vi "ModeChange.vi"(6 "DB":T1 items=["Server", "Local DB"], 7 "References":T2, 8 "error in":errorcluster, 9 "Ctrl in":refnum<vi>, 10 "Mode in":T12, 11 "Queues in":T9) -> (0 "error out":errorcluster, 2 "Mode out":T12, 3 "Queues out":T9)   [LabVIEW 2019]
uses:
  TypeDef/#TypeDef_Enum_Buttons.ctl
  Queue/TypeDef/#TypeDef_App_Queues.ctl
  TypeDef/#TypeDef_EventStructureConstant.ctl
  TypeDef/#TypeDef_Enum_EventStructure.ctl
  Queue/TypeDef/#TypeDef_NetworkStream.ctl
  Communication/TypeDef/#TypeDef_FromMRtoPC.ctl
  Communication/TypeDef/#TypeDef_FromPCtoMR.ctl
  Communication/TypeDef/#TypeDef_Command.ctl
  Communication/TypeDef/#TypeDef_ErrorHandler_prop.ctl
  Communication/TypeDef/#TypeDef_PropGraph.ctl
  Communication/TypeDef/#TypeDef_PropertiesToSave.ctl
  <vilib>/addons/database/Connection.llb/Conn ObjectReference.ctl
  Test/TypeDef/#TypeDef_DataToTest.ctl
  TypeDef/#TypeDef_References.ctl
  TypeDef/#TypeDef_Buttons.ctl
  TypeDef/#TypeDef_ReferencesMeassurementProp.ctl
  TypeDef/#TypeDef_ReferencesArchiveProp.ctl
  TypeDef/#TypeDef_Lists.ctl
  TypeDef/#TypeDef_MeasProp.ctl
  TypeDef/#TypeDef_OpProp.ctl
  TypeDef/#TypeDef_Enum_ModeOp.ctl
  Data Saving/DataBase/TypeDef/#TypeDef_DBMode.ctl
  <vilib>/addons/database/NI_Database_API.lvlib
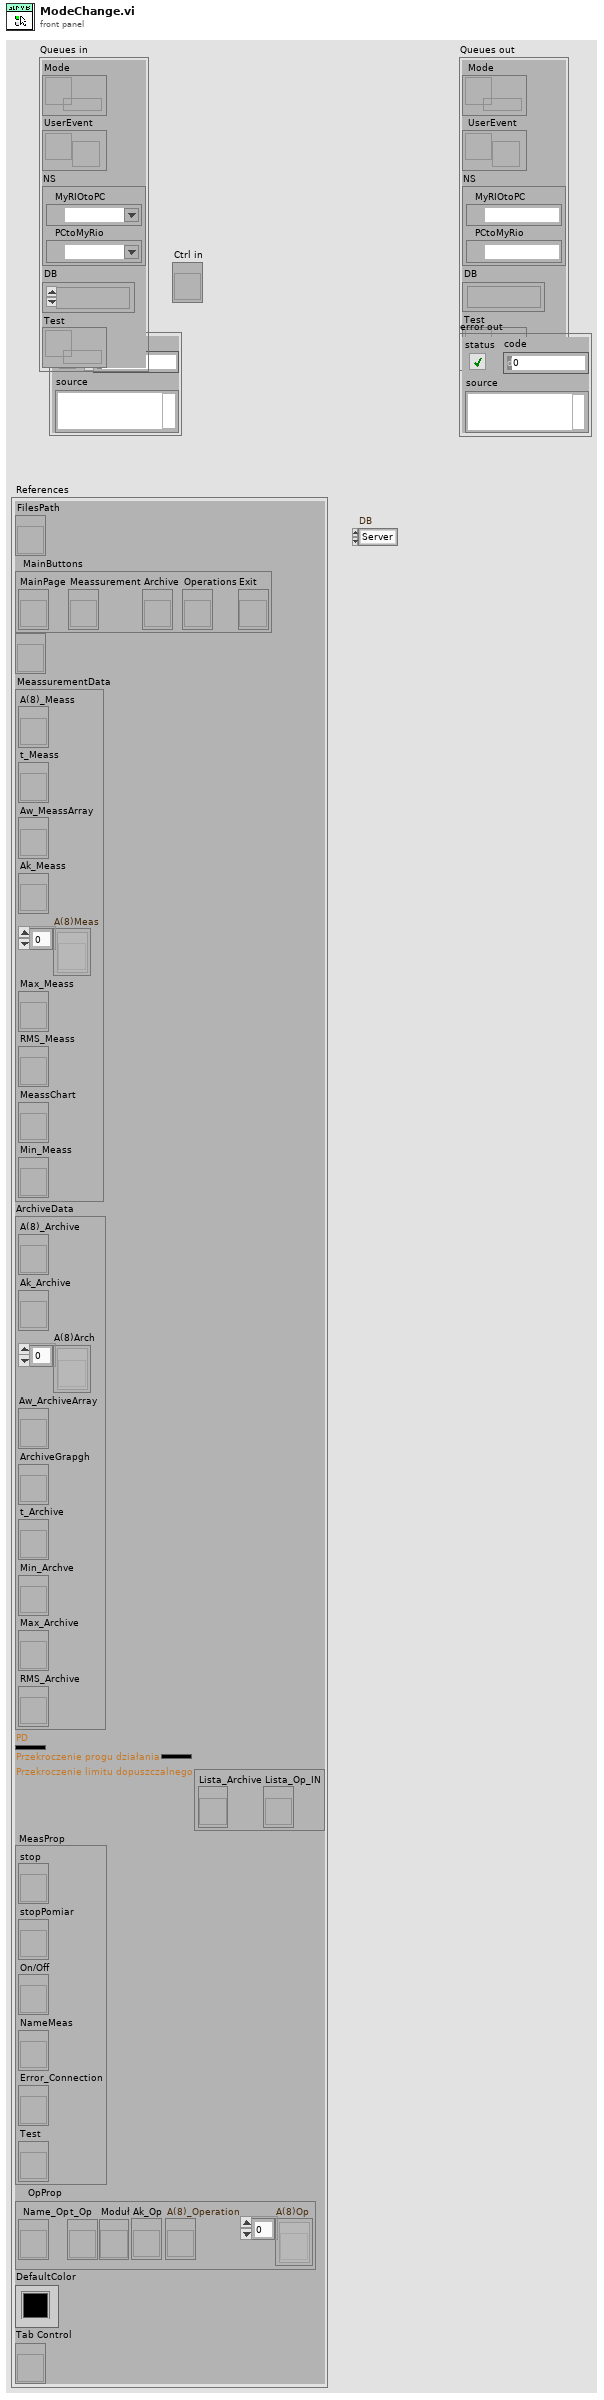
[diagram p1: front panel]
types:
  T1 = typedef "#TypeDef_DBMode.ctl" = u16
  T2 = typedef "#TypeDef_References.ctl" = cluster{"FilesPath":refnum<vi>, "MainButtons":T3, "Lista CTRL":refnum<vi>, "MeassurementData":T4, "ArchiveData":T5, "PD":u32, "LD":u32, "Lists":T6, "MeasProp":T7, "OpProp":T8, "DefaultColor":u32, "Tab Control":refnum<vi>}
  T3 = typedef "#TypeDef_Buttons.ctl" = cluster{"MainPage":refnum<vi>, "Meassurement":refnum<vi>, "Archive":refnum<vi>, "Operations":refnum<vi>, "Exit":refnum<vi>}
  T4 = typedef "#TypeDef_ReferencesMeassurementProp.ctl" = cluster{"A(8)_Meass":refnum<vi>, "t_Meass":refnum<vi>, "Aw_MeassArray":refnum<vi>, "Ak_Meass":refnum<vi>, "A(8)Meas":refnum<vi>[], "Max_Meass":refnum<vi>, "RMS_Meass":refnum<vi>, "MeassChart":refnum<vi>, "Min_Meass":refnum<vi>}
  T5 = typedef "#TypeDef_ReferencesArchiveProp.ctl" = cluster{"A(8)_Archive":refnum<vi>, "Ak_Archive":refnum<vi>, "A(8)Arch":refnum<vi>[], "Aw_ArchiveArray":refnum<vi>, "ArchiveGrapgh":refnum<vi>, "t_Archive":refnum<vi>, "Min_Archve":refnum<vi>, "Max_Archive":refnum<vi>, "RMS_Archive":refnum<vi>}
  T6 = typedef "#TypeDef_Lists.ctl" = cluster{"Lista_Archive":refnum<vi>, "Lista_Op_IN":refnum<vi>}
  T7 = typedef "#TypeDef_MeasProp.ctl" = cluster{"stop":refnum<vi>, "stopPomiar":refnum<vi>, "On/Off":refnum<vi>, "NameMeas":refnum<vi>, "Error_Connection":refnum<vi>, "Test":refnum<vi>}
  T8 = typedef "#TypeDef_OpProp.ctl" = cluster{"Name_Op":refnum<vi>, "t_Op":refnum<vi>, "Modu³":refnum<vi>, "Ak_Op":refnum<vi>, "A(8)_Operation":refnum<vi>, "A(8)Op":refnum<vi>[]}
  T9 = typedef "#TypeDef_App_Queues.ctl" = cluster{"Mode":refnum<queue>, "UserEvent":refnum<user-event>, "NS":T10, "DB":T11, "Test":refnum<queue>}
  T10 = typedef "#TypeDef_NetworkStream.ctl" = cluster{"MyRIOtoPC":refnum<k21>, "PCtoMyRio":refnum<k21>}
  T11 = typedef "NI_Database_API.lvlib/Conn ObjectReference.ctl" = refnum<k1>
  T12 = typedef "#TypeDef_Enum_Buttons.ctl" = enum32{"MainPage", "Pomiar", "Archiwum", "Operacje", "Wyjœcie"}
  T13 = typedef "#TypeDef_Enum_ModeOp.ctl" = enum16{"Oblicz ekspozycjê dzienn¹", "Uœrednij"}
  T14 = enum8{"Enabled", "Disabled", "Disabled and Grayed Out"}
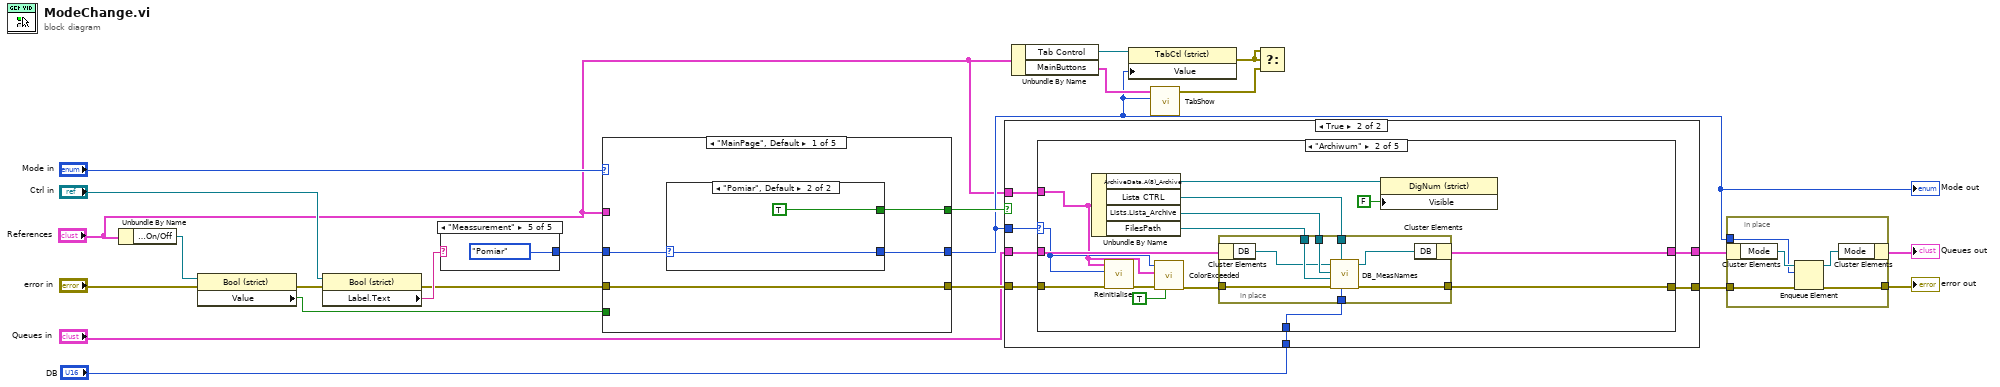
[diagram p0: block diagram]
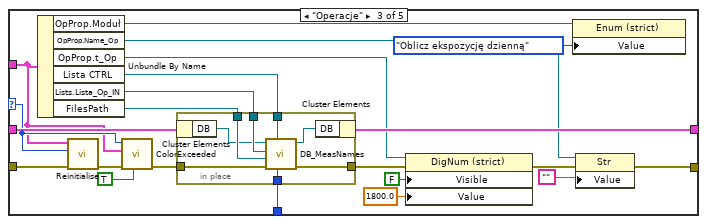
[diagram p4: hidden frame]
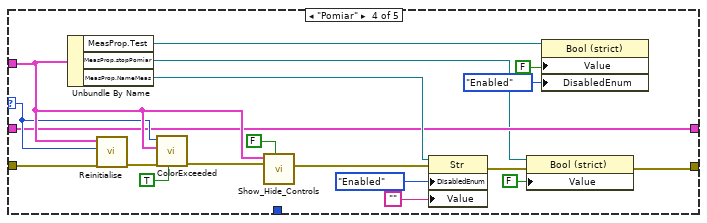
[diagram p5: hidden frame]
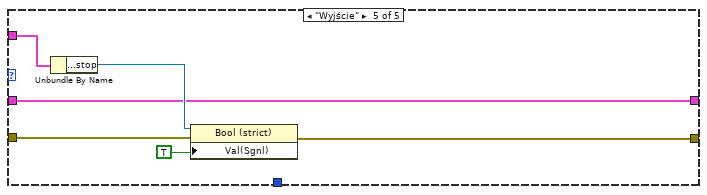
[diagram p6: hidden frame]
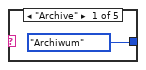
[diagram p7: hidden frame]
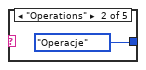
[diagram p8: hidden frame]
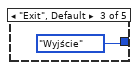
[diagram p9: hidden frame]
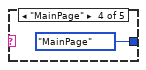
[diagram p10: hidden frame]
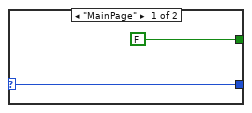
[diagram p11: hidden frame]
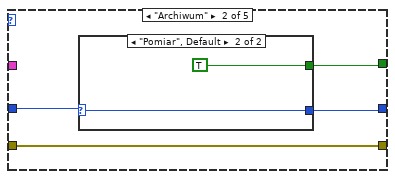
[diagram p12: hidden frame]
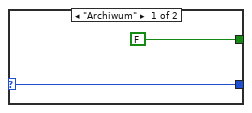
[diagram p13: hidden frame]
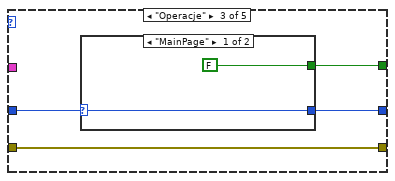
[diagram p14: hidden frame]
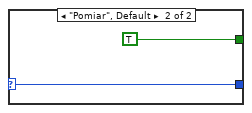
[diagram p15: hidden frame]
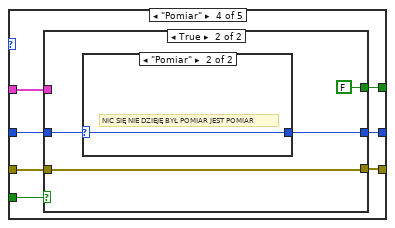
[diagram p16: hidden frame]
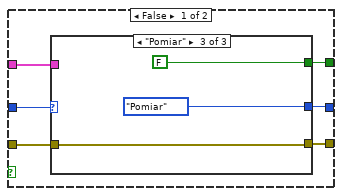
[diagram p17: hidden frame]
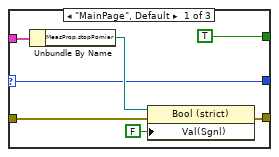
[diagram p18: hidden frame]
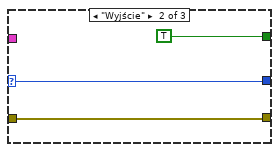
[diagram p19: hidden frame]
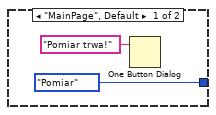
[diagram p20: hidden frame]
diagram:
  n1 = Unbundle By Name("References") -> ("MeasProp.On/Off"=w23:refnum<vi>)
  n2 = property class="Bool (strict)"(reference=w23, error in="error in") -> (error out=w21:errorcluster, "Value"=w17:bool)  [unwired: 1 out]
  n3 = property class="Bool (strict)"(reference="Ctrl in", error in=w21) -> (error out=w16:errorcluster, "Label.Text"=w19:string)  [unwired: 1 out]
  n4 = case shown="\"Meassurement\"" w19 {
    tunnel: [#TypeDef_Enum_Buttons."Archiwum" ("Value") #TypeDef_Enum_Buttons."Operacje" ("Value") #TypeDef_Enum_Buttons."Wyjœcie" ("Value") #TypeDef_Enum_Buttons."MainPage" ("Value") #TypeDef_Enum_Buttons."Pomiar" ("Value")] -> w18
    frame "Archive" {
    }
    frame "Operations" {
    }
    frame "Exit", Default {
    }
    frame "MainPage" {
    }
    frame "Meassurement" {
    }
  }
  n5 = case shown="\"MainPage\", Default" "Mode in" {
    tunnel: w18 -> [w32 w38 w47 w58 _]
    tunnel: w17 -> [_ _ _ w59 _]
    tunnel: w16 -> [w29 w37 w45 w57 w86]
    tunnel: "References" -> [_ _ _ w56 _]
    tunnel: [w31 w39 w46 w54 #TypeDef_Enum_Buttons."Wyjœcie" ("Value")] -> w5
    tunnel: [w30 w40 w48 w53 FALSE] -> w11
    tunnel: [w29 w37 w45 w55 w86] -> w10
    frame "MainPage", Default {
      n6 = case shown="\"Pomiar\", Default" w32 {
        selector: w32 -> [w34 w36]
        tunnel: [w34 w36] -> w31
        tunnel: [FALSE TRUE] -> w30
        frame "MainPage" {
        }
        frame "Pomiar", Default {
        }
      }
    }
    frame "Archiwum" {
      n7 = case shown="\"Pomiar\", Default" w38 {
        selector: w38 -> [w42 w44]
        tunnel: [w42 w44] -> w39
        tunnel: [FALSE TRUE] -> w40
        frame "Archiwum" {
        }
        frame "Pomiar", Default {
        }
      }
    }
    frame "Operacje" {
      n8 = case shown="\"MainPage\"" w47 {
        selector: w47 -> [w50 w52]
        tunnel: [w50 w52] -> w46
        tunnel: [FALSE TRUE] -> w48
        frame "MainPage" {
        }
        frame "Pomiar", Default {
        }
      }
    }
    frame "Pomiar" {
      n9 = case shown="True" w59 {
        tunnel: w58 -> [w65 w82]
        tunnel: [w64 w81] -> w54
        tunnel: w57 -> [w63 w80]
        tunnel: [w62 FALSE] -> w53
        tunnel: w56 -> [w61 _]
        tunnel: [w60 w80] -> w55
        frame False {
          n10 = case shown="\"Pomiar\"" w65 {
            selector: w65 -> [w66 w75 _]
            tunnel: [w66 w75 #TypeDef_Enum_Buttons."Pomiar" ("Value")] -> w64
            tunnel: w63 -> [w72 w73 w77]
            tunnel: [TRUE TRUE FALSE] -> w62
            tunnel: w61 -> [w70 _ _]
            tunnel: [w67 w73 w77] -> w60
            frame "MainPage", Default {
              n11 = Unbundle By Name(w70) -> ("MeasProp.stopPomiar"=w69:refnum<vi>)
              n12 = property class="Bool (strict)"(reference=w69, error in=w72, "Val(Sgnl)"=FALSE ("Value (Signaling)")) -> (error out=w67:errorcluster)  [unwired: 1 out]
            }
            frame "Wyjœcie" {
            }
            frame "Pomiar" {
            }
          }
        }
        frame True {
          n13 = case shown="\"Pomiar\"" w82 {
            selector: w82 -> [_ w85]
            tunnel: [#TypeDef_Enum_Buttons."Pomiar" ("Value") w85] -> w81
            frame "MainPage", Default {
              n14 = One Button Dialog(message="Pomiar trwa!") -> ()  [unwired: 1 in, 1 out]
            }
            frame "Pomiar" {
              # "NIC SIÊ NIE DZIEJÊ BY£ POMIAR JEST POMIAR"
            }
          }
        }
      }
    }
    frame "Wyjœcie" {
    }
  }
  "Mode out" <- w5
  n15 = case shown="True" w11 {
    tunnel: w5 -> [_ w97]
    tunnel: w10 -> [w90 w96]
    tunnel: [w90 w94] -> w9
    tunnel: "References" -> [_ w95]
    tunnel: "Queues in" -> [w89 w93]
    tunnel: [w89 w92] -> w7
    tunnel: "DB" -> [_ w91]
    frame False {
    }
    frame True {
      n16 = case shown="\"Archiwum\"" w97 {
        selector: w97 -> [_ w103 w124 w161 _]
        tunnel: w96 -> [w98 w105 w128 w166 w176]
        tunnel: w95 -> [_ w102 w123 w163 w174]
        tunnel: [w98 w114 w138 w158 w173] -> w94
        tunnel: w93 -> [w99 w108 w143 w160 w172]
        tunnel: [w99 w107 w144 w160 w172] -> w92
        tunnel: w91 -> [_ w106 w129 _ _]
        frame "MainPage", Default {
        }
        frame "Archiwum" {
          n17 = Unbundle By Name(w102) -> ("ArchiveData.A(8)_Archive"=w113:refnum<vi>, "Lista CTRL"=w111:refnum<vi>, "Lists.Lista_Archive"=w110:refnum<vi>, "FilesPath"=w109:refnum<vi>)
          n18 = call "Reinitialise.vi"("error in"=w105, "Value"=w103, "References in"=w102) -> ("error out"=w104:errorcluster)  [unwired: 8 in]
          n19 = call "ColorExceeded.vi"("Init"=TRUE, "error in"=w104, "References"=w102, "Value"=w103) -> ("error out"=w100:errorcluster)  [unwired: 7 in]
          n20 = in-place {
            in-place-border: w100 -> [w122]
            in-place-border: [w121] -> w114
            in-place-border: w111 -> [w120]
            in-place-border: w110 -> [w119]
            in-place-border: w109 -> [w118]
            in-place-border: w106 -> [w115]
            n21 = in-place-cluster #1(w108) -> ("DB"=w117:T11)
            n22 = call "DB_MeasNames.vi"("DB"=w115, "Lista pomiarów"=w120, "error in"=w122, "FilesPath"=w118, "Lista_Archive"=w119, "DB in"=w117) -> ("error out"=w121:errorcluster, "DataBase out"=w116:T11)  [unwired: 4 in]
            n23 = in-place-cluster #1("DB"=w116) -> (w107:T9)
          }
          n24 = property class="DigNum (strict)"(reference=w113, "Visible"=FALSE) -> ()  [unwired: 1 in, 2 out]
        }
        frame "Operacje" {
          n25 = Unbundle By Name(w123) -> ("OpProp.Modu³"=w134:refnum<vi>, "OpProp.Name_Op"=w132:refnum<vi>, "OpProp.t_Op"=w137:refnum<vi>, "Lista CTRL"=w140:refnum<vi>, "Lists.Lista_Op_IN"=w141:refnum<vi>, "FilesPath"=w142:refnum<vi>)
          n26 = call "Reinitialise.vi"("error in"=w128, "Value"=w124, "References in"=w123) -> ("error out"=w127:errorcluster)  [unwired: 8 in]
          n27 = call "ColorExceeded.vi"("Init"=TRUE, "error in"=w127, "References"=w123, "Value"=w124) -> ("error out"=w126:errorcluster)  [unwired: 7 in]
          n28 = in-place {
            in-place-border: w126 -> [w152]
            in-place-border: [w151] -> w139
            in-place-border: w140 -> [w150]
            in-place-border: w141 -> [w149]
            in-place-border: w142 -> [w148]
            in-place-border: w129 -> [w145]
            n29 = in-place-cluster #2(w143) -> ("DB"=w147:T11)
            n30 = call "DB_MeasNames.vi"("DB"=w145, "Lista pomiarów"=w150, "error in"=w152, "FilesPath"=w148, "Lista_Archive"=w149, "DB in"=w147) -> ("error out"=w151:errorcluster, "DataBase out"=w146:T11)  [unwired: 4 in]
            n31 = in-place-cluster #2("DB"=w146) -> (w144:T9)
          }
          n32 = property class="DigNum (strict)"(reference=w137, error in=w139, "Visible"=FALSE, "Value"=1800.0) -> (error out=w131:errorcluster)  [unwired: 1 out]
          n33 = property class="Enum (strict)"(reference=w134, "Value"=#TypeDef_Enum_ModeOp."Oblicz ekspozycjê dzienn¹") -> ()  [unwired: 1 in, 2 out]
          n34 = property class="Str"(reference=w132, error in=w131, "Value"="") -> (error out=w138:errorcluster)  [unwired: 1 out]
        }
        frame "Pomiar" {
          n35 = Unbundle By Name(w163) -> ("MeasProp.Test"=w155:refnum<vi>, "MeasProp.stopPomiar"=w157:refnum<vi>, "MeasProp.NameMeas"=w170:refnum<vi>)
          n36 = call "Reinitialise.vi"("error in"=w166, "Value"=w161, "References in"=w163) -> ("error out"=w165:errorcluster)  [unwired: 8 in]
          n37 = call "ColorExceeded.vi"("Init"=TRUE, "error in"=w165, "References"=w163, "Value"=w161) -> ("error out"=w164:errorcluster)  [unwired: 7 in]
          n38 = call "Show_Hide_Controls.vi"("Visible"=FALSE, "error in"=w164, "References"=w163) -> ("error out"=w168:errorcluster)  [unwired: 8 in]
          n39 = property class="Str"(reference=w170, error in=w168, "DisabledEnum"=T14."Enabled" ("Disabled"), "Value"="") -> (error out=w159:errorcluster)  [unwired: 1 out]
          n40 = property class="Bool (strict)"(reference=w157, error in=w159, "Value"=FALSE) -> (error out=w158:errorcluster)  [unwired: 1 out]
          n41 = property class="Bool (strict)"(reference=w155, "Value"=FALSE, "DisabledEnum"=T14."Enabled" ("Disabled")) -> ()  [unwired: 1 in, 2 out]
        }
        frame "Wyjœcie" {
          n42 = Unbundle By Name(w174) -> ("MeasProp.stop"=w175:refnum<vi>)
          n43 = property class="Bool (strict)"(reference=w175, error in=w176, "Val(Sgnl)"=TRUE ("Value (Signaling)")) -> (error out=w173:errorcluster)  [unwired: 1 out]
        }
      }
    }
  }
  n44 = Unbundle By Name("References") -> ("Tab Control"=w15:refnum<vi>, "MainButtons"=w14:T3)
  n45 = property class="TabCtl (strict)"(reference=w15, "Value"=w5) -> (error out=w13:errorcluster)  [unwired: 1 in, 1 out]
  n46 = call "TabShow.vi"("index"=w5, "Buttons"=w14) -> ("error out"=w12:errorcluster)  [unwired: 9 in]
  n47 = Select(t=w13, s=w13, f=w12) -> ()  [unwired: 1 out]
  n48 = in-place {
    in-place-border: w9 -> [w182]
    in-place-border: [w181] -> w6
    in-place-border: w5 -> [w178]
    n49 = in-place-cluster #3(w7) -> ("Mode"=w180:refnum<queue>)
    n50 = Enqueue Element(queue=w180, element=w178, error in (no error)=w182) -> (queue out=w179:refnum<queue>, error out=w181:errorcluster)  [unwired: 1 in, 1 out]
    n51 = in-place-cluster #3("Mode"=w179) -> (→"Queues out":T9)
  }
  "error out" <- w6
